vi "Create Payload (Random).vi"(7 "Bit Length":u16(ring) items=["Byte (8 bits)", "Word (16 bits)", "Long (32 bits)", "Quad (64 bits)"], 11 "Length":i32) -> (2 "Value not in range?":bool, 3 "Payload (U8)":u8[](array[numeric]) format="%.0x")   [LabVIEW 2020, in "EthFrameManagement.lvlib"]
uses:
  EthFrameManagement.lvlib
  <vilib>/numeric/Random Number (Range) U64.vi
  <vilib>/numeric/sub_Random U32.vi
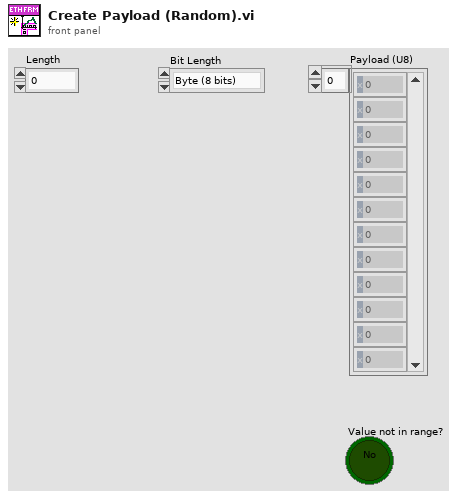
[diagram p1: front panel]
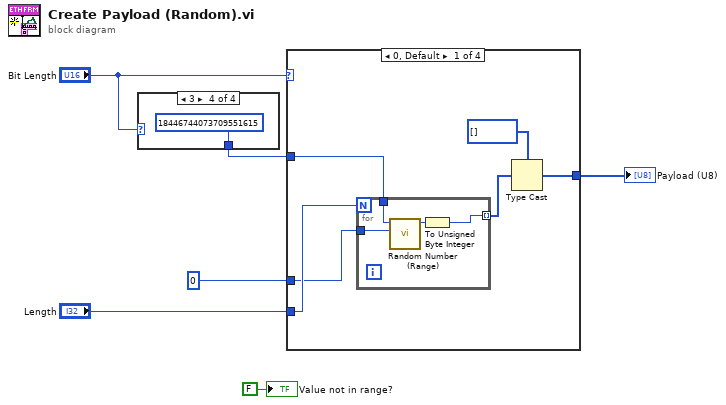
[diagram p0: block diagram]
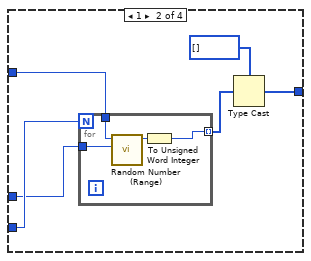
[diagram p2: hidden frame]
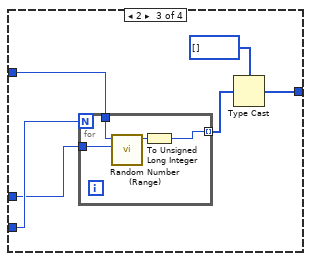
[diagram p3: hidden frame]
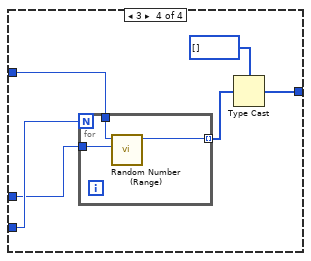
[diagram p4: hidden frame]
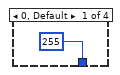
[diagram p5: hidden frame]
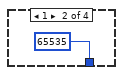
[diagram p6: hidden frame]
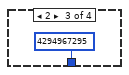
[diagram p7: hidden frame]
diagram:
  n1 = case shown="3" "Bit Length" {
    tunnel: [u64 255 ("upper limit") u64 65535 ("upper limit") u64 4294967295 ("upper limit") u64 18446744073709551615 ("upper limit")] -> w3
    frame 0, Default {
    }
    frame 1 {
    }
    frame 2 {
    }
    frame 3 {
    }
  }
  n2 = case shown="0, Default" "Bit Length" {
    tunnel: "Length" -> [w14 w24 w34 w44]
    tunnel: [w15 w25 w35 w45] -> w4
    tunnel: w3 -> [w12 w22 w32 w42]
    tunnel: u64 0 ("lower limit") -> [w11 w21 w31 w41]
    frame 0, Default {
      n3 = for {
        N: w14 -> [_]
        tunnel: [w17] -> w13 mode=indexing
        tunnel: w12 -> [w20]
        tunnel: w11 -> [w19]
        n4 = call-poly <vilib>:"Random Number (Range).vi"("lower bound (0)"=w19, "upper bound (100)"=w20) -> ("number"=w18:u64)  [unwired: 9 in]
        n5 = To Unsigned Byte Integer(number=w18) -> (unsigned 8bit integer=w17:u8)
      }
      n6 = Type Cast(type=u8[] [] ("Array"), x=w13) -> (*(type *) &x=w15:u8[])
    }
    frame 1 {
      n7 = for {
        N: w24 -> [_]
        tunnel: [w27] -> w23 mode=indexing
        tunnel: w22 -> [w30]
        tunnel: w21 -> [w29]
        n8 = call-poly <vilib>:"Random Number (Range).vi"("lower bound (0)"=w29, "upper bound (100)"=w30) -> ("number"=w28:u64)  [unwired: 9 in]
        n9 = To Unsigned Word Integer(number=w28) -> (unsigned 16bit integer=w27:u16)
      }
      n10 = Type Cast(type=u8[] [] ("Array"), x=w23) -> (*(type *) &x=w25:u8[])
    }
    frame 2 {
      n11 = for {
        N: w34 -> [_]
        tunnel: [w37] -> w33 mode=indexing
        tunnel: w32 -> [w40]
        tunnel: w31 -> [w39]
        n12 = call-poly <vilib>:"Random Number (Range).vi"("lower bound (0)"=w39, "upper bound (100)"=w40) -> ("number"=w38:u64)  [unwired: 9 in]
        n13 = To Unsigned Long Integer(number=w38) -> (unsigned 32bit integer=w37:u32)
      }
      n14 = Type Cast(type=u8[] [] ("Array"), x=w33) -> (*(type *) &x=w35:u8[])
    }
    frame 3 {
      n15 = for {
        N: w44 -> [_]
        tunnel: [w47] -> w43 mode=indexing
        tunnel: w42 -> [w49]
        tunnel: w41 -> [w48]
        n16 = call-poly <vilib>:"Random Number (Range).vi"("lower bound (0)"=w48, "upper bound (100)"=w49) -> ("number"=w47:u64)  [unwired: 9 in]
      }
      n17 = Type Cast(type=u8[] [] ("Array"), x=w43) -> (*(type *) &x=w45:u8[])
    }
  }
  "Payload (U8)" <- w4
  "Value not in range?" <- FALSE ("Value not in range?")
